vi "SelectOPCTags.LoadOPCTree.vi"(8 "error in (no error)":errorcluster, 9 "Connection.Properties":T1={"Server IP Address"="localhost", "Server Port"=49350, "Message Mode"=enum."None", "Security"=enum."Basic256", "User Name"="", "Password"="", "Client Certificate"=path "", "Server Certificate"=path "", "Server Certificate (RT)"=path "", "Client Certificate (RT)"=path ""}, 10 "Tree":refnum<vi>, 11 "VI in":refnum<vi>) -> (0 "error out":errorcluster, 3 "LUT":variant)   [LabVIEW 2019, in "OPC UA Client Addon System Explorer.lvlib"]
uses:
  OPC UA Client Addon System Explorer.lvlib
  Addon Shared/Types/OPCConnection.Properties.ctl
  <vilib>/OPCUA/NI OPC UA Client.lvlib
  Addon Shared/OPC UA Client Addon Shared.lvlib
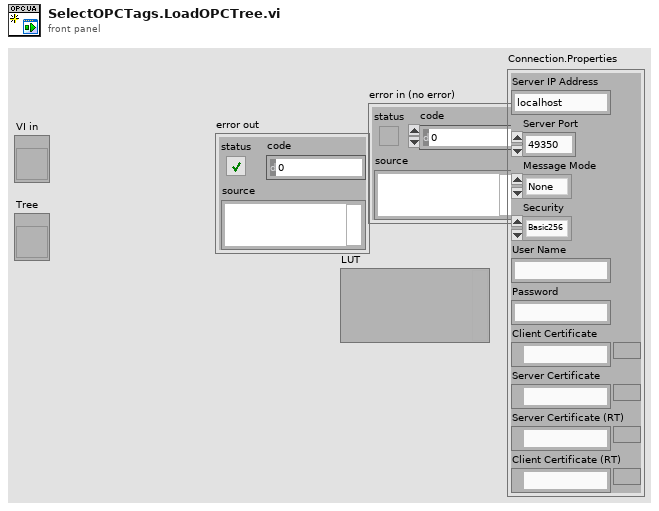
[diagram p1: front panel]
types:
  T1 = typedef "OPC UA Client Addon Shared.lvlib/OPCConnection.Properties.ctl" = cluster{"Server IP Address":string, "Server Port":u16, "Message Mode":enum16{"None", "Sign", "Sign and Encrypt"}, "Security":enum16{"Basic256", "Basic128Rsa15"}, "User Name":string, "Password":string, "Client Certificate":path, "Server Certificate":path, "Server Certificate (RT)":path, "Client Certificate (RT)":path}
  T2 = cluster{"message mode":enum16{"None", "Sign", "Sign and Encrypt"}, "security":enum16{"Basic256", "Basic128Rsa15"}}
  T3 = typedef "OPC UA Client Refnum.ctl" = refnum<k21>
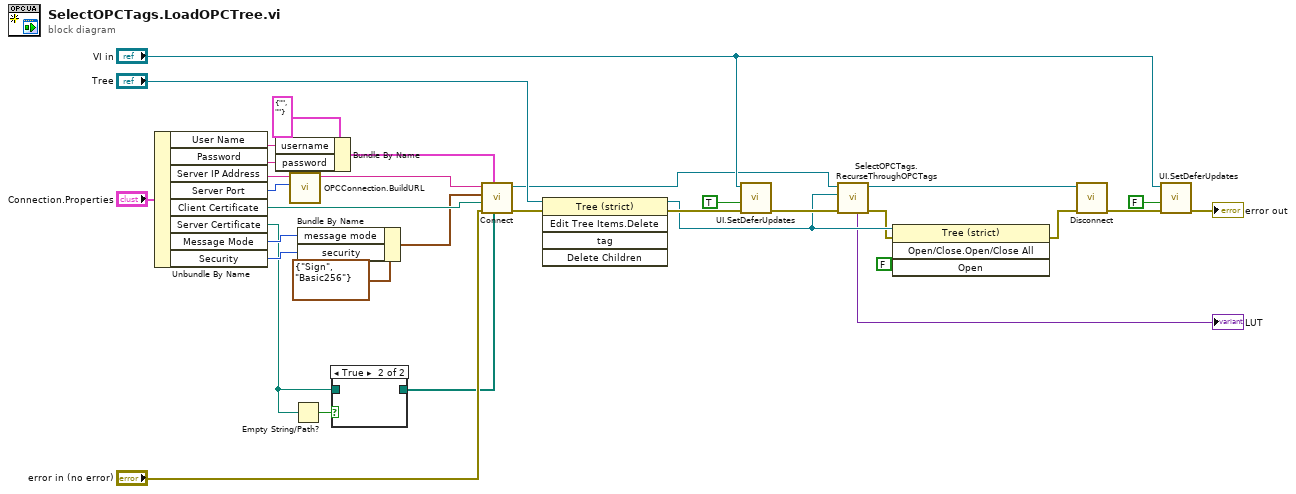
[diagram p0: block diagram]
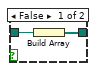
[diagram p2: hidden frame]
diagram:
  n1 = Unbundle By Name("Connection.Properties") -> ("User Name"=w14:string, "Password"=w15:string, "Server IP Address"=w18:string, "Server Port"=w17:u16, "Client Certificate"=w11:path, "Server Certificate"=w2:path, "Message Mode"=w8:enum16{"None", "Sign", "Sign and Encrypt"}, "Security"=w7:enum16{"Basic256", "Basic128Rsa15"})
  n2 = Bundle By Name(cluster=cluster{"username":string, "password":string} {"username"="", "password"=""} ("username/password"), "username"=w14, "password"=w15) -> (w12:cluster{"username":string, "password":string})
  n3 = call "OPCConnection.BuildURL.vi"("Server Port"=w17, "Server IP Address"=w18) -> ("OPC Path"=w16:string)  [unwired: 9 in]
  n4 = Empty String/Path?(string/path=w2) -> (empty?=w3:bool)
  n5 = Bundle By Name(cluster=T2 {"message mode"=enum."Sign", "security"=enum."Basic256"} ("security policy"), "message mode"=w8, "security"=w7) -> (w9:T2)
  n6 = case shown="True" w3 {
    tunnel: [w35 _] -> w1
    tunnel: w2 -> [w34 _]
    frame False {
      n7 = Build Array(w34) -> (w35:path[])
    }
    frame True {
    }
  }
  n8 = call <vilib>:"Connect.vi"("trusted server certificates"=w1, "username/password"=w12, "error in (no error)"="error in (no error)", "client certificate file"=w11, "security policy"=w9, "server endpoint URL"=w16) -> ("error out"=w5:errorcluster, "OPC UA client refnum out"=w4:T3)  [unwired: 3 in, 1 out]
  n9 = invoke class="Tree (strict)" method="Edit Tree Items.Delete"(reference="Tree", error in=w5) -> (reference out=w26:refnum<vi>, error out=w32:errorcluster)  [unwired: 3 in, 3 out]
  n10 = call "UI.SetDeferUpdates.vi"("error in (no error)"=w32, "Defer Panel Updates"=TRUE, "This VI"="VI in") -> ("error out"=w33:errorcluster)  [unwired: 8 in]
  n11 = call "SelectOPCTags.RecurseThroughOPCTags.vi"("error in (no error)"=w33, "reference out"=w26, "OPC UA Client Ref"=w4) -> ("error out"=w24:errorcluster, "OPC UA Client Ref"=w22:refnum<k21>, "LUT"=→"LUT":variant)  [unwired: 6 in]
  n12 = invoke class="Tree (strict)" method="Open/Close.Open/Close All"(reference=w26, error in=w24, "Open"=FALSE ("Open?")) -> (error out=w25:errorcluster)  [unwired: 1 in, 3 out]
  n13 = call <vilib>:"Disconnect.vi"("error in (no error)"=w25, "OPC UA client refnum in"=w22) -> ("error out"=w29:errorcluster)  [unwired: 9 in]
  n14 = call "UI.SetDeferUpdates.vi"("error in (no error)"=w29, "Defer Panel Updates"=FALSE, "This VI"="VI in") -> ("error out"=→"error out":errorcluster)  [unwired: 8 in]
